vi "Shutdown.vi"(8 "error in (no error)":errorcluster, 11 "FRTS Process in":refnum<class "FRTS Process.lvclass">) -> (0 "error out":errorcluster)   [LabVIEW 2019, in "TimingDRV Engine.lvlib" / "FRTS Process.lvclass"]
uses:
  FRTS Process.lvclass
  C:/Users/XEnderMD/Desktop/CD Project Tools/Source/Engine/Parent Classes/Process/Process.lvclass
  Parent Classes/Process/Process.lvclass/Process.ctl
  FRTS Process.lvclass/FRTS Process.ctl
  <vilib>/NI VeriStand/Custom Device API/Get Item Property (String).vi
  Parent Classes/Process/Process.lvclass
  Parent Classes/TimerDRV Class/TimerDRV.lvclass
  <vilib>/NI VeriStand/Custom Device API/Custom Device API.lvlib
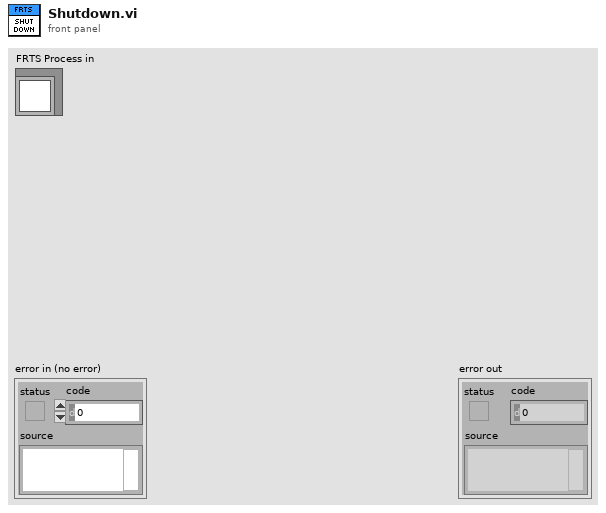
[diagram p1: front panel]
types:
  T1 = typedef "TimingDRV Engine.lvlib/Process.lvclass/Async Paramters.ctl" = cluster{"Device Reference":T2, "Device Clock":string, "Device Inputs FIFO":refnum<k33>, "Device Outputs FIFO":refnum<k33>, "CD Engine Event Ref":T3}
  T2 = typedef "Custom Device API.lvlib/Custom Device Item Ref.ctl" = u64
  T3 = typedef "Custom Device API.lvlib/Custom Device Engine Event Ref.ctl" = refnum<event-registration>
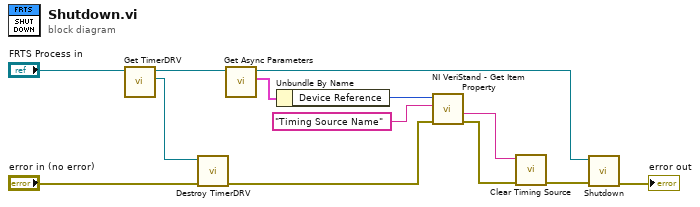
[diagram p0: block diagram]
diagram:
  n1 = call "Get TimerDRV.vi"("FRTS Process in"="FRTS Process in") -> ("TimingDRV Engine.lvlib:TimerDRV.lvclass"=w10:refnum<class "TimerDRV.lvclass">, "FRTS Process out"=w9:refnum<class "FRTS Process.lvclass">)  [unwired: 9 in]
  n2 = call "Destroy TimerDRV.vi"("error in (no error)"="error in (no error)", "TimerDRV in"=w10) -> ("error out"=w6:errorcluster)  [unwired: 9 in]
  n3 = call "Get Async Parameters.vi"("Process in"=w9) -> ("Async Parameters"=w8:T1, "Process out"=w1:refnum<class "FRTS Process.lvclass">)  [unwired: 9 in]
  n4 = Unbundle By Name(w8) -> ("Device Reference"=w7:T2)
  n5 = call-poly <vilib>:"NI VeriStand - Get Item Property.vi"("error in (no error)"=w6, "Property Name"="Timing Source Name", "Item Ref in"=w7) -> ("error out"=w3:errorcluster, "Value"=w4:string)  [unwired: 5 in, 2 out]
  n6 = call <vilib>:"Clear Timing Source.vi"("error in (no error)"=w3, "name"=w4) -> ("error out"=w2:errorcluster)  [unwired: 8 in, 1 out]
  n7 = call-parent "Shutdown.vi"("error in (no error)"=w2, "Process in"=w1) -> ("error out"=→"error out":errorcluster)  [unwired: 9 in]
